vi "NT Read Variant.vi"(4 "options":T1={"Send All"=FALSE, "Keep Duplicates"=FALSE, "rate (hz)"=10}, 8 "error in":errorcluster, 9 "default value":variant, 11 "name":string="Variant") -> (0 "error out":errorcluster, 3 "Variant":variant)   [LabVIEW 2025]
doc: "Return the variant stored in the named topic. Returns an error and the default value if topic not present."
uses:
  <vilib>/Rock Robotics/Network Tables/NT SubscribeOptions.ctl
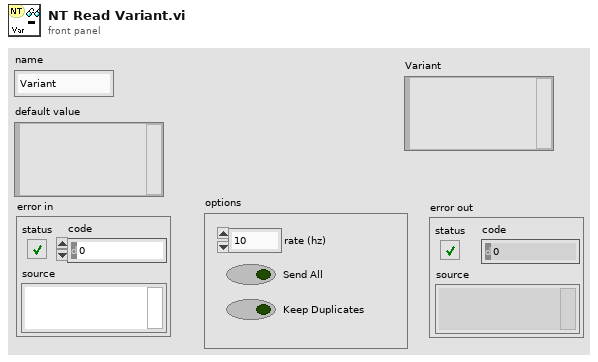
[diagram p1: front panel]
types:
  T1 = typedef "NT SubscribeOptions.ctl" = cluster{"Send All":bool, "Keep Duplicates":bool, "rate (hz)":u64}
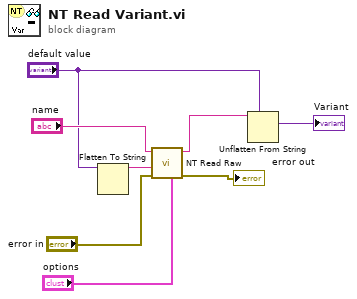
[diagram p0: block diagram]
diagram:
  n1 = Flatten To String(anything="default value") -> (data string=w2:string)  [unwired: 3 in, 2 out]
  n2 = call <vilib>:"NT Read Raw.vi"("options"="options", "error in"="error in", "default value"=w2, "name"="name") -> ("error out"=→"error out":errorcluster, "raw"=w4:string)  [unwired: 6 in]
  n3 = Unflatten From String(type="default value", binary string=w4) -> (value=→"Variant":variant)  [unwired: 3 in, 2 out]
